vi "CRYRub & Buzz Loudness Global.vi"() -> ()   [LabVIEW 2013]
panel:
  in  "Rub & Buzz Total":dbl=44100.0
  in  "pre-final Loudness":dbl=44100.0
  in  "Rub &Buzz NL":dbl=44100.0
  in  "Rub & Buzz Fe":dbl=44100.0
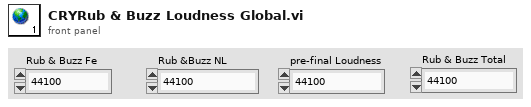
[diagram p1: front panel]
diagram:
